vi "Interface - Header.vi"(7 "Msg Chain":string, 8 "error in (no error)":errorcluster {"code" format="Error %.0f"}, 10 "Interfaces":refnum<class "Interface Documenation.lvclass">[](array[class]), 11 "VIDoc Printer - Confluence In":refnum<class "VIDoc Printer - Confluence.lvclass">) -> (0 "error out":errorcluster {"code" format="Error %.0f"}, 3 "VIDoc Printer - Confluence Out":refnum<class "VIDoc Printer - Confluence.lvclass">)   [LabVIEW 2023, in "VIDoc Printer - Confluence.lvlib" / "VIDoc Printer - Confluence.lvclass"]
uses:
  VIDoc Printer - Confluence.lvclass
  C:/projects/DMC/Tooling/Git-Action-Service/Source/Documentation Generation/Printers/Printer/VIDoc Printer.lvclass
  Parsing/Interface Documenation/Interface Documenation.lvclass
  Confluence Formatting/Types/Format Combo Box.ctl
  Parsing/Interface Documenation/Interface Documenation.lvclass/Interface Documenation.ctl
  Parsing/Interface Documenation/Get Name.vi
  Parsing/Interface Documenation/Get Qualified Name.vi
  VIDoc Printer - Confluence.lvclass/VIDoc Printer - Confluence.ctl
  Printer/VIDoc Printer.lvclass
  UI Interaction/UI Interaction.lvclass
  Confluence Formatting/Confluence Formatting.lvlib
  C:/projects/DMC/Tooling/Git-Action-Service/Source/Documentation Generation/Printers/Confluence Printer/VIDoc Printer - Confluence.lvclass
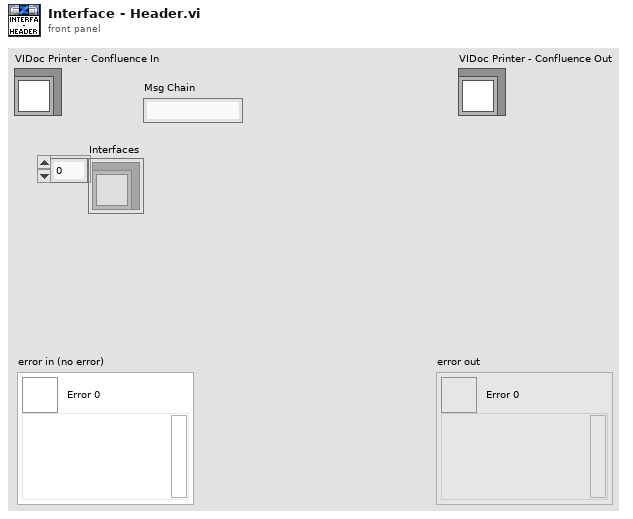
[diagram p1: front panel]
types:
  T1 = typedef "Confluence Formatting.lvlib/Format Combo Box.ctl" = string
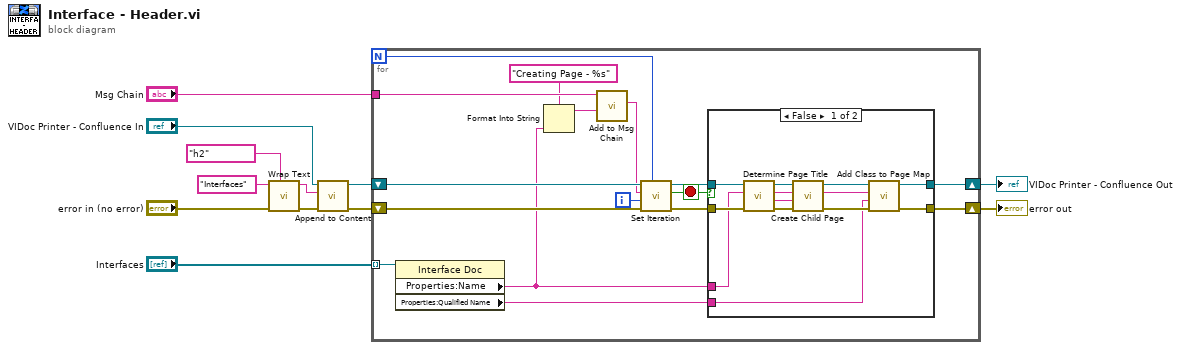
[diagram p0: block diagram]
diagram:
  n1 = call "Wrap Text.vi"("Formatting"=T1 "h2", "Error in"="error in (no error)", "String"="Interfaces") -> ("Error out"=w11:errorcluster, "Wrapped String"=w10:string)  [unwired: 7 in]
  n2 = call "Append to Content.vi"("error in (no error)"=w11, "Content"=w10, "VIDoc Printer - Confluence In"="VIDoc Printer - Confluence In") -> ("error out"=w8:errorcluster, "VIDoc Printer - Confluence Out"=w7:refnum<class "VIDoc Printer - Confluence.lvclass">)  [unwired: 7 in]
  n3 = for {
    N -> [w21]
    shift-right: [w27] -> w5
    shift-left: w7 -> [w25]
    shift-right: [w28] -> w6
    shift-left: w8 -> [w24]
    tunnel: "Interfaces" -> [w26] mode=indexing
    tunnel: "Msg Chain" -> [w19]
    i -> [w20]
    stop <- w14 stop-if-true
    n4 = property class="Interface Doc"(reference=w26) -> ("Properties:Name"=w15:string, "Properties:Qualified Name"=w13:string)  [unwired: 1 in, 2 out]
    n5 = Format Into String(format string="Creating Page - %s", w15) -> (resulting string=w17:string)  [unwired: 2 in, 1 out]
    n6 = call "Add to Msg Chain.vi"("New"=w17, "Msg Chain in"=w19) -> ("Msg Chain out"=w16:string)  [unwired: 9 in]
    n7 = call "Set Iteration.vi"("Progress Max"=w21, "error in (no error)"=w24, "Progress Value"=w20, "Message (No Message Update)"=w16, "VIDoc Printer In"=w25) -> ("error out"=w22:errorcluster, "Abort?"=w14:bool, "VIDoc Printer Out"=w23:refnum<class "VIDoc Printer - Confluence.lvclass">)  [unwired: 4 in]
    n8 = case shown="False" w14 {
      tunnel: [w31 w41] -> w28
      tunnel: [w33 w40] -> w27
      tunnel: w23 -> [w39 w40]
      tunnel: w22 -> [w38 w41]
      tunnel: w15 -> [w36 _]
      tunnel: w13 -> [w29 _]
      frame False {
        n9 = call "Determine Page Title.vi"("error in (no error)"=w38, "Name"=w36, "VIDoc Printer - Confluence In"=w39) -> ("error out"=w37:errorcluster, "Parent Page Title"=w35:string, "Page Title"=w30:string)  [unwired: 5 in, 1 out]
        n10 = call "Create Child Page.vi"("error in (no error)"=w37, "Parent Page Title"=w35, "New Page Title"=w30, "VIDoc Printer - Confluence In"=w39) -> ("error out"=w32:errorcluster, "VIDoc Printer - Confluence Out"=w34:refnum<class "VIDoc Printer - Confluence.lvclass">)  [unwired: 5 in, 1 out]
        n11 = call "Add Class to Page Map.vi"("error in (no error)"=w32, "Class Qualified Name"=w29, "Page Name"=w30, "VIDoc Printer - Confluence In"=w34) -> ("error out"=w31:errorcluster, "VIDoc Printer - Confluence Out"=w33:refnum<class "VIDoc Printer - Confluence.lvclass">)  [unwired: 6 in]
      }
      frame True {
      }
    }
  }
  "error out" <- w6
  "VIDoc Printer - Confluence Out" <- w5
